vi "Read 2D Picture.vi"(8 "error in (no error)":errorcluster, 11 "class2 in":refnum<class "class2.lvclass">) -> (0 "error out":errorcluster, 2 "2D Picture":picture, 3 "class2 out":refnum<class "class2.lvclass">)   [LabVIEW 2013, in "class2.lvclass"]
uses:
  class2.lvclass
  class2.lvclass/class2.ctl
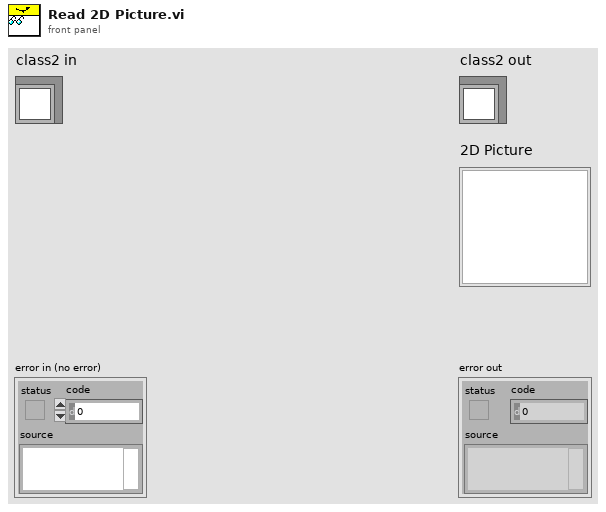
[diagram p1: front panel]
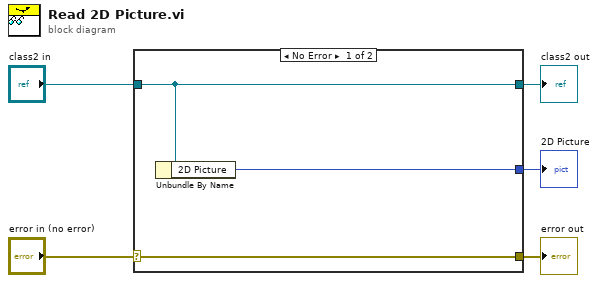
[diagram p0: block diagram]
diagram:
  n1 = case shown="No Error" "error in (no error)" {
    selector: "error in (no error)" -> [w8 w9]
    tunnel: [w8 w9] -> w4
    tunnel: [w7 w10] -> w2
    tunnel: "class2 in" -> [w7 w10]
    tunnel: [w6 _] -> w1
    frame No Error {
      n2 = Unbundle By Name(w7) -> ("2D Picture"=w6:picture)
    }
    frame Error {
    }
  }
  "error out" <- w4
  "class2 out" <- w2
  "2D Picture" <- w1
